vi "XPS_LTA_HS_Jogger.vi"(4 "Axis 2":string="Group3", 5 "Axis 1":string="Group2", 7 "Controller Address":string="192.168.254.254") -> ()   [LabVIEW 2016]
panel:
  in  "stop 2":bool
  in  "Refresh Time\n(msec)":u32=100 min=50 max=10000 step=1
  out "Axis 2 position":dbl format="%.10f"
  out "Axis 1 position":dbl format="%.10f"
  out "Axis 2 Status":string
  out "Axis 1 Status":string
  in  "Velocity (slow)\nmm/s":dbl=1.0 min=0.0 max=5.0
  in  "Velocity (fast)\nmm/s":dbl=5.0 min=0.0 max=5.0
  in  "Fast motion parameter":T1={"Velocity (units/s)"=5.0, "Acceleration (units/s²)"=20.0} {"Acceleration (units/s²)" format="%.6f"; "Velocity (units/s)" format="%.6f"}
  in  "Axis 2 Positive fast":bool
  in  "Axis 2 Positive":bool
  in  "Axis 2 negative fast":bool
  in  "Axis 2 negative":bool
  in  "Axis 1 Positive fast":bool
  in  "Axis 1 Positive":bool
  in  "Axis 1 negative fast":bool
  in  "Axis 1 negative":bool
  in  "Slow motion parameter":T1={"Velocity (units/s)"=1.0, "Acceleration (units/s²)"=20.0} {"Acceleration (units/s²)" format="%.6f"; "Velocity (units/s)" format="%.6f"}
  in  "stop":bool
  # "1"
  # "2"
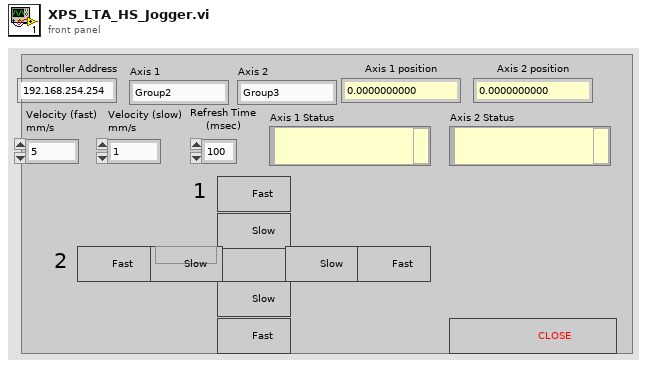
[diagram p1: front panel]
types:
  T1 = cluster{"Velocity (units/s)":dbl, "Acceleration (units/s²)":dbl}
  T2 = cluster{"connection TCP":refnum<k5>, "LogTo File":bool, "Log File refnum":refnum<file>, "no error if error log":bool}
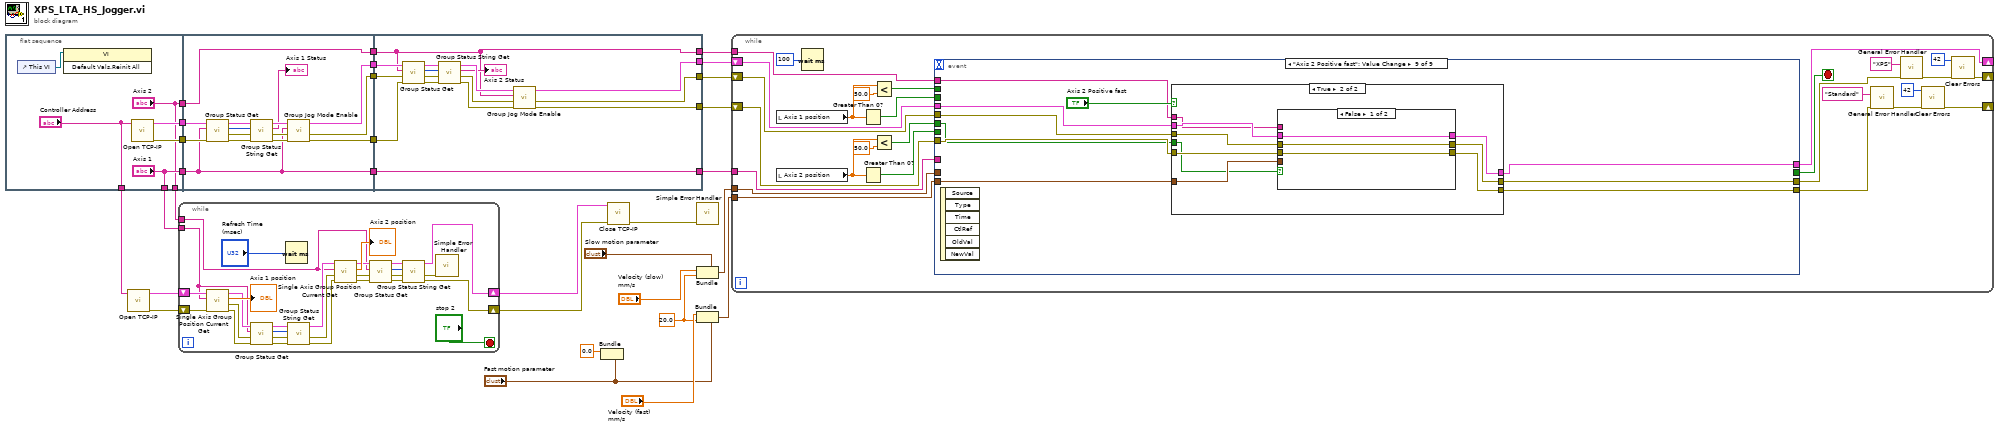
[diagram p0: block diagram]
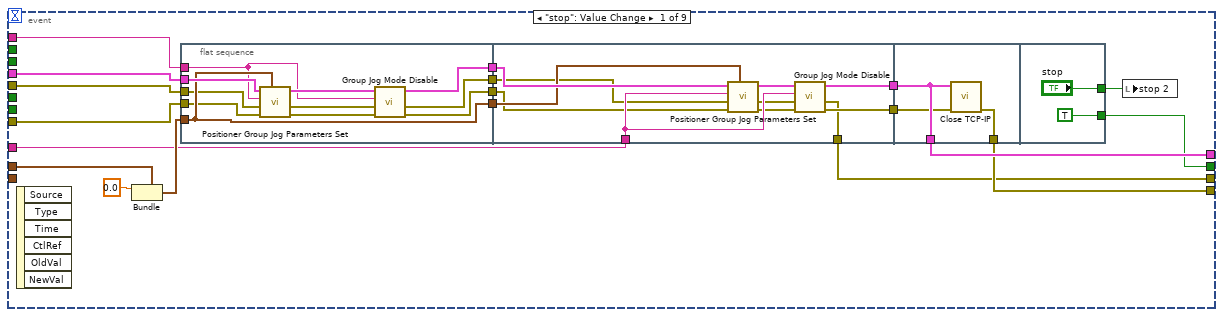
[diagram p2: hidden frame]
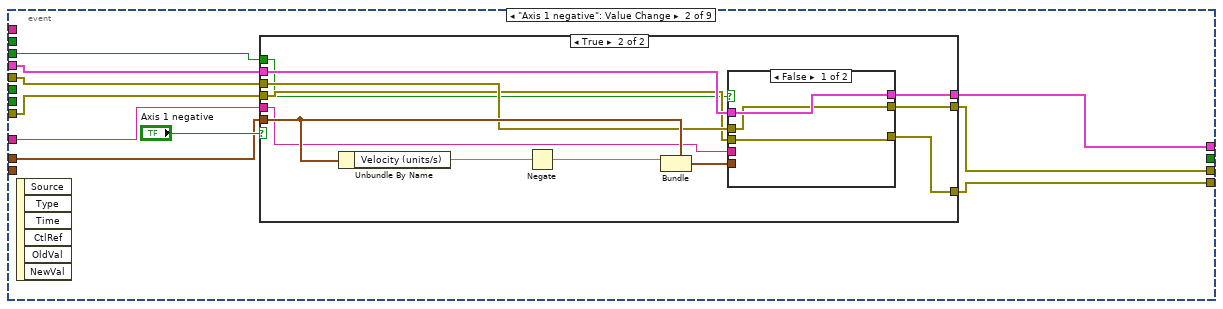
[diagram p3: hidden frame]
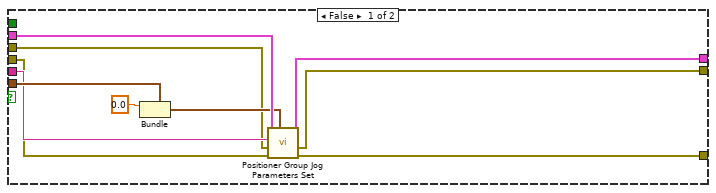
[diagram p4: hidden frame]
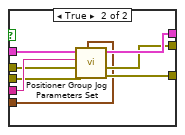
[diagram p5: hidden frame]
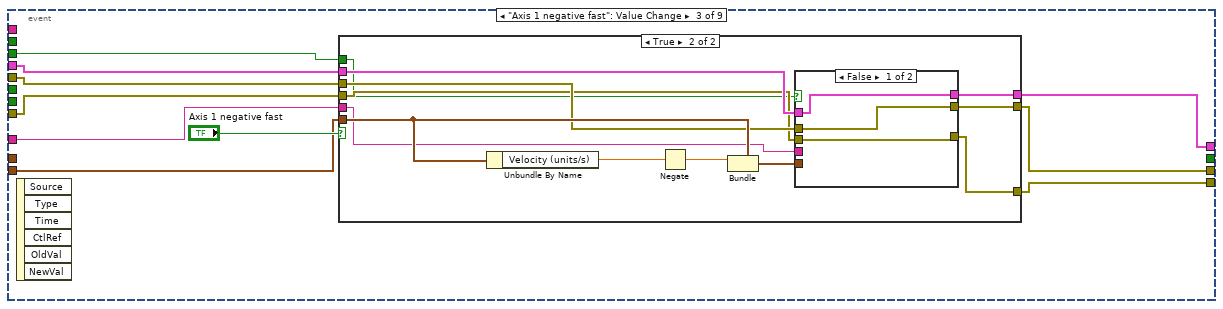
[diagram p6: hidden frame]
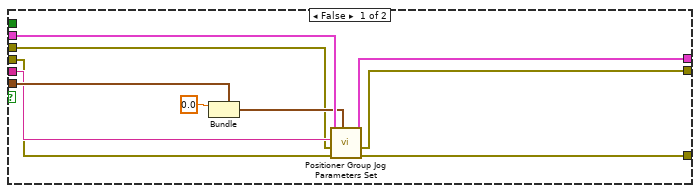
[diagram p7: hidden frame]
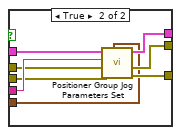
[diagram p8: hidden frame]
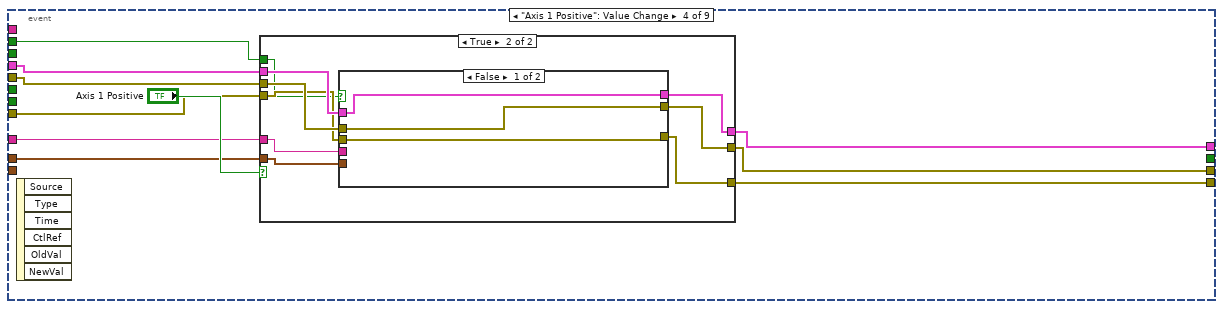
[diagram p9: hidden frame]
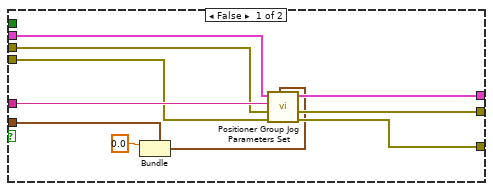
[diagram p10: hidden frame]
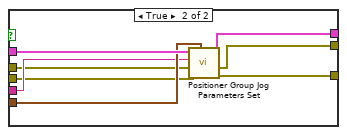
[diagram p11: hidden frame]
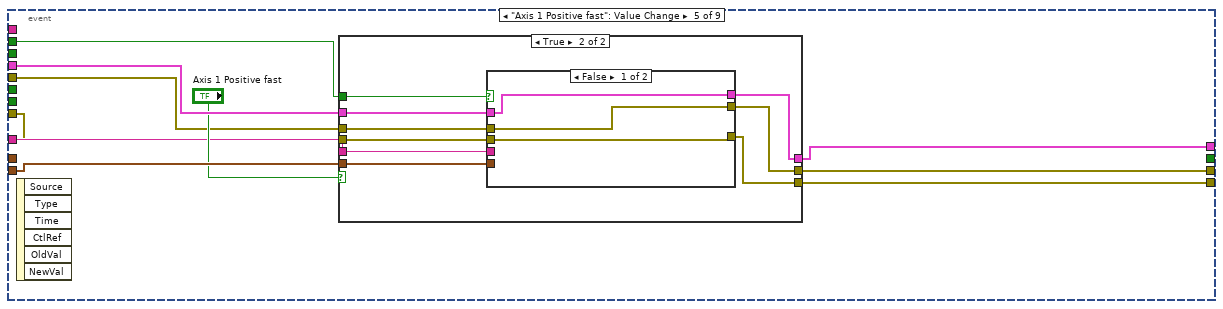
[diagram p12: hidden frame]
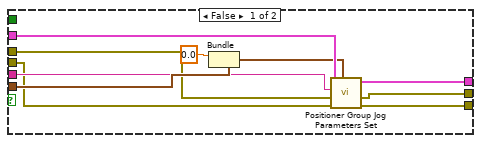
[diagram p13: hidden frame]
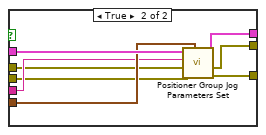
[diagram p14: hidden frame]
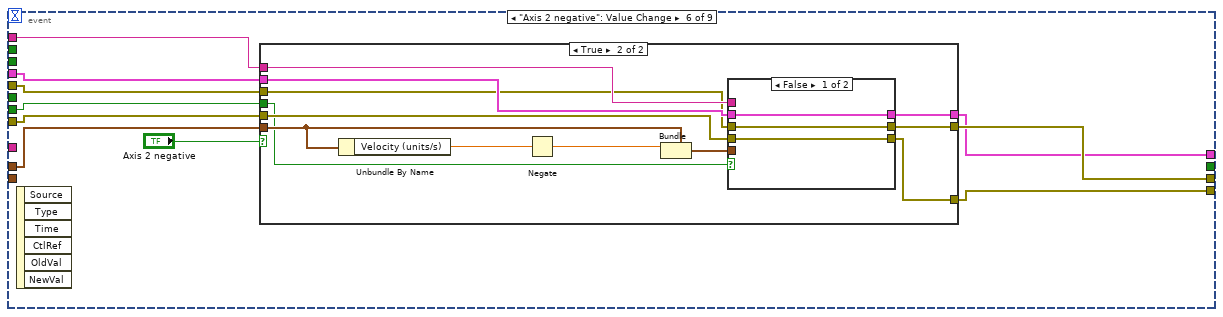
[diagram p15: hidden frame]
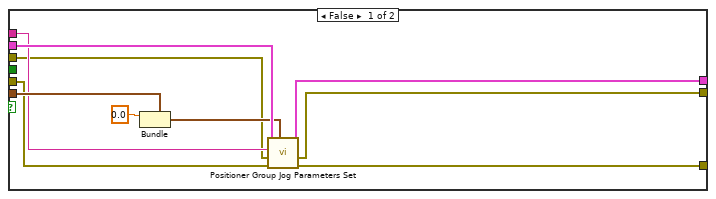
[diagram p16: hidden frame]
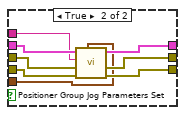
[diagram p17: hidden frame]
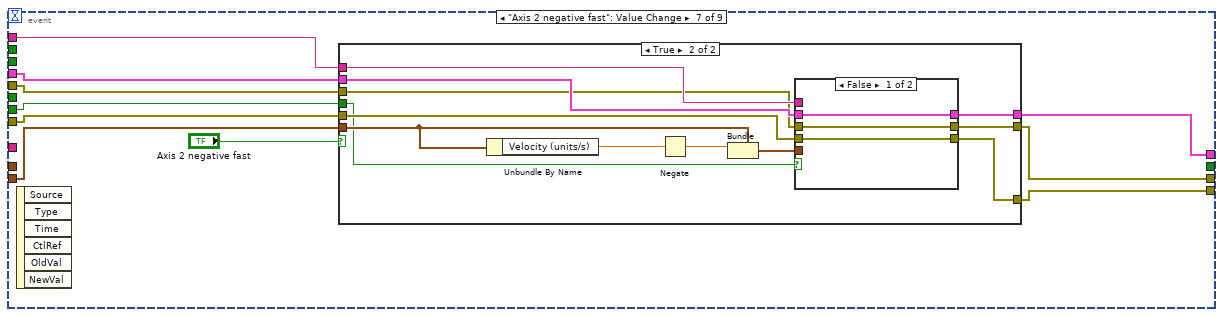
[diagram p18: hidden frame]
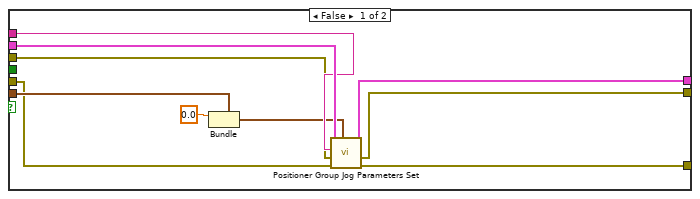
[diagram p19: hidden frame]
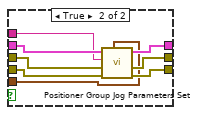
[diagram p20: hidden frame]
diagram:
  w22 = 20.0 ("Acceleration (units/s²)")
  n1 = flat-sequence {
    tunnel: ["Axis 1"] -> w19
    tunnel: [w35] -> w18
    tunnel: [w34] -> w17
    tunnel: ["Axis 2"] -> w16
    tunnel: ["Controller Address"] -> w10
    tunnel: ["Axis 1"] -> w5
    tunnel: ["Axis 2"] -> w4
    tunnel: [w51] -> w30
    tunnel: [w50] -> w29
    tunnel: [w49] -> w28
    tunnel: w19 -> [w37]
    tunnel: w18 -> [w44]
    tunnel: w17 -> [w43]
    tunnel: w16 -> [w38]
    tunnel: [w38] -> w15
    tunnel: [w37] -> w13
    tunnel: w30 -> [w64]
    tunnel: w29 -> [w58]
    tunnel: w28 -> [w59]
    tunnel: w15 -> [w53]
    tunnel: w13 -> [w54]
    tunnel: [w57] -> w2
    tunnel: [w56] -> w14
    tunnel: [w54] -> w11
    tunnel: [w53] -> w12
    tunnel: [w52] -> w1
    frame #0 {
      n2 = control-ref of="This VI"() -> (w36:refnum<vi>)
      n3 = invoke class="VI" method="Default Vals.Reinit All"(reference=w36) -> ()  [unwired: 2 in, 3 out]
      n4 = call <userlib>:"Open TCP-IP.vi"("IP address"="Controller Address") -> ("error out"=w35:errorcluster, "Connection ID"=w34:T2)  [unwired: 5 in, 4 out]
    }
    frame #1 {
      n5 = call <userlib>:"Group Status Get.vi"("error in (no error)"=w44, "Group Name (250 c max)"=w37, "connection ID in"=w43) -> ("error out"=w47:errorcluster, "XPS error out"=w48:errorcluster, "Status"=w46:i32, "connection ID out"=w42:T2)  [unwired: 5 in]
      n6 = call <userlib>:"Group Status String Get.vi"("error in (no error)"=w47, "XPS error in (no error)"=w48, "Status #"=w46, "connection ID in"=w42) -> ("error out"=w41:errorcluster, "XPS error out"=w40:errorcluster, "Group Status String"=→"Axis 1 Status":string, "connection ID out"=w45:T2)  [unwired: 4 in]
      n7 = call <userlib>:"Group Jog Mode Enable.vi"("error in (no error)"=w41, "XPS error in (no error)"=w40, "Group Name (250 c max)"=w37, "connection ID in"=w45) -> ("error out"=w49:errorcluster, "XPS error out"=w50:errorcluster, "connection ID out"=w51:T2)  [unwired: 5 in]
    }
    frame #2 {
      n8 = call <userlib>:"Group Status Get.vi"("error in (no error)"=w59, "XPS error in (no error)"=w58, "Group Name (250 c max)"=w53, "connection ID in"=w64) -> ("error out"=w66:errorcluster, "XPS error out"=w67:errorcluster, "Status"=w65:i32, "connection ID out"=w63:T2)  [unwired: 4 in]
      n9 = call <userlib>:"Group Status String Get.vi"("error in (no error)"=w66, "XPS error in (no error)"=w67, "Status #"=w65, "connection ID in"=w63) -> ("error out"=w61:errorcluster, "XPS error out"=w60:errorcluster, "Group Status String"=→"Axis 2 Status":string, "connection ID out"=w62:T2)  [unwired: 4 in]
      n10 = call <userlib>:"Group Jog Mode Enable.vi"("error in (no error)"=w61, "XPS error in (no error)"=w60, "Group Name (250 c max)"=w53, "connection ID in"=w62) -> ("error out"=w52:errorcluster, "XPS error out"=w57:errorcluster, "connection ID out"=w56:T2)  [unwired: 5 in]
    }
  }
  n11 = call <userlib>:"Open TCP-IP.vi"("IP address"=w10) -> ("error out"=w8:errorcluster, "Connection ID"=w9:T2)  [unwired: 5 in, 4 out]
  n12 = while {
    shift-right: [w70] -> w7
    shift-left: w9 -> [w95]
    shift-right: [w69] -> w6
    shift-left: w8 -> [w94]
    tunnel: w5 -> [w86]
    tunnel: w4 -> [w73]
    stop <- "stop 2" stop-if-true
    n13 = call <userlib>:"Single Axis Group Position Current Get.vi"("error in (no error)"=w94, "SingleAxis Group  Name (250 c max)"=w86, "connection ID in"=w95) -> ("error out"=w85:errorcluster, "XPS error out"=w84:errorcluster, "Current Position (units)"=→"Axis 1 position":dbl, "connection ID out"=w89:T2)  [unwired: 5 in]
    n14 = call <userlib>:"Group Status Get.vi"("error in (no error)"=w85, "XPS error in (no error)"=w84, "Group Name (250 c max)"=w86, "connection ID in"=w89) -> ("error out"=w82:errorcluster, "XPS error out"=w83:errorcluster, "Status"=w87:i32, "connection ID out"=w88:T2)  [unwired: 4 in]
    n15 = Wait (ms)(milliseconds to wait="Refresh Time\n(msec)") -> ()  [unwired: 1 out]
    n16 = call <userlib>:"Group Status String Get.vi"("error in (no error)"=w82, "XPS error in (no error)"=w83, "Status #"=w87, "connection ID in"=w88) -> ("error out"=w79:errorcluster, "XPS error out"=w80:errorcluster, "connection ID out"=w81:T2)  [unwired: 4 in, 1 out]
    n17 = call <userlib>:"Single Axis Group Position Current Get.vi"("error in (no error)"=w79, "XPS error in (no error)"=w80, "SingleAxis Group  Name (250 c max)"=w73, "connection ID in"=w81) -> ("error out"=w76:errorcluster, "XPS error out"=w77:errorcluster, "Current Position (units)"=→"Axis 2 position":dbl, "connection ID out"=w78:T2)  [unwired: 4 in]
    n18 = call <userlib>:"Group Status Get.vi"("error in (no error)"=w76, "XPS error in (no error)"=w77, "Group Name (250 c max)"=w73, "connection ID in"=w78) -> ("error out"=w74:errorcluster, "XPS error out"=w75:errorcluster, "Status"=w71:i32, "connection ID out"=w72:T2)  [unwired: 4 in]
    n19 = call <userlib>:"Group Status String Get.vi"("error in (no error)"=w74, "XPS error in (no error)"=w75, "Status #"=w71, "connection ID in"=w72) -> ("error out"=w69:errorcluster, "XPS error out"=w68:errorcluster, "connection ID out"=w70:T2)  [unwired: 4 in, 1 out]
    n20 = call <vilib>:"Simple Error Handler.vi"("error in (no error)"=w68) -> ()  [unwired: 4 in, 5 out]
  }
  n21 = Bundle(cluster="Fast motion parameter", "Velocity (units/s)"=0.0) -> ()  [unwired: 1 in, 1 out]
  n22 = call <userlib>:"Close TCP-IP.vi"("error in (no error)"=w6, "connection ID in"=w7) -> ("Error out"=w3:errorcluster)  [unwired: 9 in]
  n23 = call <vilib>:"Simple Error Handler.vi"("error in (no error)"=w3) -> ()  [unwired: 4 in, 5 out]
  n24 = Bundle(cluster="Slow motion parameter", "Velocity (units/s)"="Velocity (slow)\nmm/s", "Acceleration (units/s²)"=w22) -> (w24:T1)
  n25 = Bundle(cluster="Fast motion parameter", "Velocity (units/s)"="Velocity (fast)\nmm/s", "Acceleration (units/s²)"=w22) -> (w27:T1)
  n26 = while {
    shift-right: [w122] -> _
    shift-left: w14 -> [w123]
    tunnel: w27 -> [w121]
    tunnel: w24 -> [w120]
    tunnel: w12 -> [w119]
    tunnel: w11 -> [w118]
    shift-right: [w96] -> _
    shift-left: w1 -> [w107]
    shift-right: [w99] -> _
    shift-left: w2 -> [w108]
    stop <- w114 stop-if-true
    n27 = local read "Axis 1 position"() -> (w110:dbl)
    n28 = local read "Axis 2 position"() -> (w109:dbl)
    n29 = Wait (ms)(milliseconds to wait=u32 100) -> ()  [unwired: 1 out]
    n30 = Greater Than 0?(x=w110) -> (x > 0?=w106:bool)
    n31 = Greater Than 0?(x=w109) -> (x > 0?=w104:bool)
    n32 = Less?(x=w110, y=50.0) -> (x < y?=w105:bool)
    n33 = Less?(x=w109, y=50.0) -> (x < y?=w103:bool)
    n34 = event shown="[8] \"Axis 2 Positive fast\": Value Change" {
      selector: _ -> [_ _ _ _ _ _ _ _ _]
      dyn-events: _ -> [_ _ _ _ _ _ _ _ _]
      timeout: _ -> [_ _ _ _ _ _ _ _ _]
      tunnel: [w125 w175 w218 w261 w304 w341 w383 w426 w466] -> w115
      tunnel: w123 -> [w142 w178 w221 w264 w305 w343 w386 w429 w470]
      tunnel: [w141 w177 w220 w263 w302 w340 w385 w428 w468] -> w122
      tunnel: [w124 w176 w219 w262 w303 w342 w384 w427 w467] -> w116
      tunnel: w121 -> [_ _ w217 _ w301 _ w387 _ w469]
      tunnel: w120 -> [w137 w174 _ w260 _ w344 _ w430 _]
      tunnel: w119 -> [w134 _ _ _ _ w339 w382 w425 w465]
      tunnel: w118 -> [w133 w173 w216 w259 w299 _ _ _ _]
      tunnel: [w132 _ _ _ _ _ _ _ _] -> w114
      tunnel: w108 -> [w130 w172 w215 w258 w298 w338 w381 w424 w464]
      tunnel: w107 -> [w126 w171 w214 w257 w297 w337 w380 w423 w463]
      tunnel: w106 -> [_ w170 w213 _ _ _ _ _ _]
      tunnel: w105 -> [_ _ _ w256 w296 _ _ _ _]
      tunnel: w104 -> [_ _ _ _ _ w336 w379 _ _]
      tunnel: w103 -> [_ _ _ _ _ _ _ w422 w462]
      event "stop": Value Change {
        n35 = event-data() -> ()  [unwired: 1 in, 6 out]
        n36 = Bundle(cluster=w137, "Velocity (units/s)"=0.0) -> (w136:T1)  [unwired: 1 in]
        n37 = flat-sequence {
          tunnel: w142 -> [w152]
          tunnel: [w151] -> w139
          tunnel: w136 -> [w150]
          tunnel: [w150] -> w135
          tunnel: w134 -> [w149]
          tunnel: w130 -> [w148]
          tunnel: [w146] -> w129
          tunnel: [w145] -> w127
          tunnel: w126 -> [w143]
          tunnel: [w162] -> w140
          tunnel: w139 -> [w164]
          tunnel: w135 -> [w161]
          tunnel: w133 -> [w160]
          tunnel: w129 -> [w159]
          tunnel: [w157] -> w128
          tunnel: w127 -> [w155]
          tunnel: [w154] -> w124
          tunnel: [w167] -> w141
          tunnel: w140 -> [w167]
          tunnel: w128 -> [w166]
          tunnel: [w165] -> w125
          tunnel: [TRUE] -> w132
          tunnel: ["stop"] -> w131
          frame #0 {
            n38 = call <userlib>:"Positioner Group Jog Parameters Set.vi"("Group Jog parameters"=w150, "error in (no error)"=w143, "XPS error in (no error)"=w148, "Positioner Name (250 c max)"=w149, "connection ID in"=w152) -> ("error out"=w144:errorcluster, "XPS error out"=w147:errorcluster, "connection ID out"=w153:T2)  [unwired: 4 in]
            n39 = call <userlib>:"Group Jog Mode Disable.vi"("error in (no error)"=w144, "XPS error in (no error)"=w147, "Group Name (250 c max)"=w149, "connection ID in"=w153) -> ("error out"=w145:errorcluster, "XPS error out"=w146:errorcluster, "connection ID out"=w151:T2)  [unwired: 5 in]
          }
          frame #1 {
            n40 = call <userlib>:"Positioner Group Jog Parameters Set.vi"("Group Jog parameters"=w161, "error in (no error)"=w155, "XPS error in (no error)"=w159, "Positioner Name (250 c max)"=w160, "connection ID in"=w164) -> ("error out"=w156:errorcluster, "XPS error out"=w158:errorcluster, "connection ID out"=w163:T2)  [unwired: 4 in]
            n41 = call <userlib>:"Group Jog Mode Disable.vi"("error in (no error)"=w156, "XPS error in (no error)"=w158, "Group Name (250 c max)"=w160, "connection ID in"=w163) -> ("error out"=w157:errorcluster, "XPS error out"=w154:errorcluster, "connection ID out"=w162:T2)  [unwired: 5 in]
          }
          frame #2 {
            n42 = call <userlib>:"Close TCP-IP.vi"("error in (no error)"=w166, "connection ID in"=w167) -> ("Error out"=w165:errorcluster)  [unwired: 9 in]
          }
          frame #3 {
          }
        }
        n43 = local write "stop 2"(w131) -> ()
      }
      event "Axis 1 negative": Value Change {
        n44 = event-data() -> ()  [unwired: 1 in, 6 out]
        n45 = case shown="True" "Axis 1 negative" {
          tunnel: w178 -> [w188 w201]
          tunnel: [w187 w199] -> w177
          tunnel: [w186 w198] -> w176
          tunnel: [w185 w197] -> w175
          tunnel: w174 -> [w189 w200]
          tunnel: w173 -> [w184 w196]
          tunnel: w172 -> [w181 w192]
          tunnel: w171 -> [w180 w191]
          tunnel: w170 -> [_ w190]
          frame False {
            n46 = Bundle(cluster=w189, "Velocity (units/s)"=0.0) -> (w182:T1)  [unwired: 1 in]
            n47 = call <userlib>:"Positioner Group Jog Parameters Set.vi"("Group Jog parameters"=w182, "error in (no error)"=w180, "XPS error in (no error)"=w181, "Positioner Name (250 c max)"=w184, "connection ID in"=w188) -> ("error out"=w185:errorcluster, "XPS error out"=w186:errorcluster, "connection ID out"=w187:T2)  [unwired: 4 in]
          }
          frame True {
            n48 = Unbundle By Name(w200) -> ("Velocity (units/s)"=w195:dbl)
            n49 = Negate(x=w195) -> (-x=w194:dbl)
            n50 = Bundle(cluster=w200, "Velocity (units/s)"=w194) -> (w193:T1)  [unwired: 1 in]
            n51 = case shown="False" w190 {
              tunnel: w201 -> [w204 w212]
              tunnel: [w204 w211] -> w199
              tunnel: [w203 w210] -> w198
              tunnel: [w202 w209] -> w197
              tunnel: w196 -> [_ w208]
              tunnel: w193 -> [_ w207]
              tunnel: w192 -> [w203 w206]
              tunnel: w191 -> [w202 w205]
              frame False {
              }
              frame True {
                n52 = call <userlib>:"Positioner Group Jog Parameters Set.vi"("Group Jog parameters"=w207, "error in (no error)"=w205, "XPS error in (no error)"=w206, "Positioner Name (250 c max)"=w208, "connection ID in"=w212) -> ("error out"=w209:errorcluster, "XPS error out"=w210:errorcluster, "connection ID out"=w211:T2)  [unwired: 4 in]
              }
            }
          }
        }
      }
      event "Axis 1 negative fast": Value Change {
        n53 = event-data() -> ()  [unwired: 1 in, 6 out]
        n54 = case shown="True" "Axis 1 negative fast" {
          tunnel: w221 -> [w231 w244]
          tunnel: [w230 w242] -> w220
          tunnel: [w229 w241] -> w219
          tunnel: [w228 w240] -> w218
          tunnel: w217 -> [w232 w243]
          tunnel: w216 -> [w227 w239]
          tunnel: w215 -> [w224 w235]
          tunnel: w214 -> [w223 w234]
          tunnel: w213 -> [_ w233]
          frame False {
            n55 = Bundle(cluster=w232, "Velocity (units/s)"=0.0) -> (w225:T1)  [unwired: 1 in]
            n56 = call <userlib>:"Positioner Group Jog Parameters Set.vi"("Group Jog parameters"=w225, "error in (no error)"=w223, "XPS error in (no error)"=w224, "Positioner Name (250 c max)"=w227, "connection ID in"=w231) -> ("error out"=w228:errorcluster, "XPS error out"=w229:errorcluster, "connection ID out"=w230:T2)  [unwired: 4 in]
          }
          frame True {
            n57 = Unbundle By Name(w243) -> ("Velocity (units/s)"=w238:dbl)
            n58 = Negate(x=w238) -> (-x=w237:dbl)
            n59 = Bundle(cluster=w243, "Velocity (units/s)"=w237) -> (w236:T1)  [unwired: 1 in]
            n60 = case shown="False" w233 {
              tunnel: w244 -> [w245 w255]
              tunnel: [w245 w254] -> w242
              tunnel: [w246 w253] -> w241
              tunnel: [w247 w252] -> w240
              tunnel: w239 -> [_ w251]
              tunnel: w236 -> [_ w250]
              tunnel: w235 -> [w246 w249]
              tunnel: w234 -> [w247 w248]
              frame False {
              }
              frame True {
                n61 = call <userlib>:"Positioner Group Jog Parameters Set.vi"("Group Jog parameters"=w250, "error in (no error)"=w248, "XPS error in (no error)"=w249, "Positioner Name (250 c max)"=w251, "connection ID in"=w255) -> ("error out"=w252:errorcluster, "XPS error out"=w253:errorcluster, "connection ID out"=w254:T2)  [unwired: 4 in]
              }
            }
          }
        }
      }
      event "Axis 1 Positive": Value Change {
        n62 = event-data() -> ()  [unwired: 1 in, 6 out]
        n63 = case shown="True" "Axis 1 Positive" {
          tunnel: w264 -> [w275 w284]
          tunnel: [w273 w282] -> w263
          tunnel: [w272 w281] -> w262
          tunnel: [w271 w280] -> w261
          tunnel: w260 -> [w274 w283]
          tunnel: w259 -> [w270 w279]
          tunnel: w258 -> [w267 w278]
          tunnel: w257 -> [w266 w277]
          tunnel: w256 -> [_ w276]
          frame False {
            n64 = Bundle(cluster=w274, "Velocity (units/s)"=0.0) -> (w268:T1)  [unwired: 1 in]
            n65 = call <userlib>:"Positioner Group Jog Parameters Set.vi"("Group Jog parameters"=w268, "error in (no error)"=w266, "XPS error in (no error)"=w267, "Positioner Name (250 c max)"=w270, "connection ID in"=w275) -> ("error out"=w271:errorcluster, "XPS error out"=w272:errorcluster, "connection ID out"=w273:T2)  [unwired: 4 in]
          }
          frame True {
            n66 = case shown="False" w276 {
              tunnel: w284 -> [w285 w295]
              tunnel: w283 -> [_ w294]
              tunnel: [w285 w293] -> w282
              tunnel: [w287 w292] -> w281
              tunnel: [w286 w291] -> w280
              tunnel: w279 -> [_ w290]
              tunnel: w278 -> [w287 w289]
              tunnel: w277 -> [w286 w288]
              frame False {
              }
              frame True {
                n67 = call <userlib>:"Positioner Group Jog Parameters Set.vi"("Group Jog parameters"=w294, "error in (no error)"=w288, "XPS error in (no error)"=w289, "Positioner Name (250 c max)"=w290, "connection ID in"=w295) -> ("error out"=w291:errorcluster, "XPS error out"=w292:errorcluster, "connection ID out"=w293:T2)  [unwired: 4 in]
              }
            }
          }
        }
      }
      event "Axis 1 Positive fast": Value Change {
        n68 = event-data() -> ()  [unwired: 1 in, 6 out]
        n69 = case shown="True" "Axis 1 Positive fast" {
          tunnel: w305 -> [w315 w324]
          tunnel: [w311 w320] -> w304
          tunnel: [w312 w321] -> w303
          tunnel: [w313 w322] -> w302
          tunnel: w301 -> [w314 w323]
          tunnel: w299 -> [w310 w319]
          tunnel: w298 -> [w307 w317]
          tunnel: w297 -> [w306 w318]
          tunnel: w296 -> [_ w316]
          frame False {
            n70 = Bundle(cluster=w314, "Velocity (units/s)"=0.0) -> (w308:T1)  [unwired: 1 in]
            n71 = call <userlib>:"Positioner Group Jog Parameters Set.vi"("Group Jog parameters"=w308, "error in (no error)"=w306, "XPS error in (no error)"=w307, "Positioner Name (250 c max)"=w310, "connection ID in"=w315) -> ("error out"=w311:errorcluster, "XPS error out"=w312:errorcluster, "connection ID out"=w313:T2)  [unwired: 4 in]
          }
          frame True {
            n72 = case shown="False" w316 {
              tunnel: w324 -> [w325 w335]
              tunnel: w323 -> [_ w334]
              tunnel: [w325 w333] -> w322
              tunnel: [w327 w332] -> w321
              tunnel: [w326 w331] -> w320
              tunnel: w319 -> [_ w330]
              tunnel: w318 -> [w326 w329]
              tunnel: w317 -> [w327 w328]
              frame False {
              }
              frame True {
                n73 = call <userlib>:"Positioner Group Jog Parameters Set.vi"("Group Jog parameters"=w334, "error in (no error)"=w329, "XPS error in (no error)"=w328, "Positioner Name (250 c max)"=w330, "connection ID in"=w335) -> ("error out"=w331:errorcluster, "XPS error out"=w332:errorcluster, "connection ID out"=w333:T2)  [unwired: 4 in]
              }
            }
          }
        }
      }
      event "Axis 2 negative": Value Change {
        n74 = event-data() -> ()  [unwired: 1 in, 6 out]
        n75 = case shown="True" "Axis 2 negative" {
          tunnel: w344 -> [w354 w367]
          tunnel: w343 -> [w355 w366]
          tunnel: [w352 w364] -> w342
          tunnel: [w351 w363] -> w341
          tunnel: [w353 w365] -> w340
          tunnel: w339 -> [w350 w362]
          tunnel: w338 -> [w347 w358]
          tunnel: w337 -> [w346 w357]
          tunnel: w336 -> [_ w356]
          frame False {
            n76 = Bundle(cluster=w354, "Velocity (units/s)"=0.0) -> (w348:T1)  [unwired: 1 in]
            n77 = call <userlib>:"Positioner Group Jog Parameters Set.vi"("Group Jog parameters"=w348, "error in (no error)"=w346, "XPS error in (no error)"=w347, "Positioner Name (250 c max)"=w350, "connection ID in"=w355) -> ("error out"=w351:errorcluster, "XPS error out"=w352:errorcluster, "connection ID out"=w353:T2)  [unwired: 4 in]
          }
          frame True {
            n78 = Unbundle By Name(w367) -> ("Velocity (units/s)"=w361:dbl)
            n79 = Negate(x=w361) -> (-x=w360:dbl)
            n80 = Bundle(cluster=w367, "Velocity (units/s)"=w360) -> (w359:T1)  [unwired: 1 in]
            n81 = case shown="False" w356 {
              tunnel: w366 -> [w370 w378]
              tunnel: [w370 w377] -> w365
              tunnel: [w369 w376] -> w364
              tunnel: [w368 w375] -> w363
              tunnel: w362 -> [_ w374]
              tunnel: w359 -> [_ w373]
              tunnel: w358 -> [w369 w372]
              tunnel: w357 -> [w368 w371]
              frame False {
              }
              frame True {
                n82 = call <userlib>:"Positioner Group Jog Parameters Set.vi"("Group Jog parameters"=w373, "error in (no error)"=w371, "XPS error in (no error)"=w372, "Positioner Name (250 c max)"=w374, "connection ID in"=w378) -> ("error out"=w375:errorcluster, "XPS error out"=w376:errorcluster, "connection ID out"=w377:T2)  [unwired: 4 in]
              }
            }
          }
        }
      }
      event "Axis 2 negative fast": Value Change {
        n83 = event-data() -> ()  [unwired: 1 in, 6 out]
        n84 = case shown="True" "Axis 2 negative fast" {
          tunnel: w387 -> [w397 w410]
          tunnel: w386 -> [w398 w409]
          tunnel: [w396 w408] -> w385
          tunnel: [w395 w407] -> w384
          tunnel: [w394 w406] -> w383
          tunnel: w382 -> [w393 w405]
          tunnel: w381 -> [w390 w401]
          tunnel: w380 -> [w389 w400]
          tunnel: w379 -> [_ w399]
          frame False {
            n85 = Bundle(cluster=w397, "Velocity (units/s)"=0.0) -> (w391:T1)  [unwired: 1 in]
            n86 = call <userlib>:"Positioner Group Jog Parameters Set.vi"("Group Jog parameters"=w391, "error in (no error)"=w389, "XPS error in (no error)"=w390, "Positioner Name (250 c max)"=w393, "connection ID in"=w398) -> ("error out"=w394:errorcluster, "XPS error out"=w395:errorcluster, "connection ID out"=w396:T2)  [unwired: 4 in]
          }
          frame True {
            n87 = Unbundle By Name(w410) -> ("Velocity (units/s)"=w404:dbl)
            n88 = Negate(x=w404) -> (-x=w403:dbl)
            n89 = Bundle(cluster=w410, "Velocity (units/s)"=w403) -> (w402:T1)  [unwired: 1 in]
            n90 = case shown="False" w399 {
              tunnel: w409 -> [w413 w421]
              tunnel: [w413 w420] -> w408
              tunnel: [w412 w419] -> w407
              tunnel: [w411 w418] -> w406
              tunnel: w405 -> [_ w417]
              tunnel: w402 -> [_ w416]
              tunnel: w401 -> [w412 w415]
              tunnel: w400 -> [w411 w414]
              frame False {
              }
              frame True {
                n91 = call <userlib>:"Positioner Group Jog Parameters Set.vi"("Group Jog parameters"=w416, "error in (no error)"=w414, "XPS error in (no error)"=w415, "Positioner Name (250 c max)"=w417, "connection ID in"=w421) -> ("error out"=w418:errorcluster, "XPS error out"=w419:errorcluster, "connection ID out"=w420:T2)  [unwired: 4 in]
              }
            }
          }
        }
      }
      event "Axis 2 Positive": Value Change {
        n92 = event-data() -> ()  [unwired: 1 in, 6 out]
        n93 = case shown="True" "Axis 2 Positive" {
          tunnel: w430 -> [w440 w449]
          tunnel: w429 -> [w441 w450]
          tunnel: [w439 w448] -> w428
          tunnel: [w438 w447] -> w427
          tunnel: [w437 w446] -> w426
          tunnel: w425 -> [w436 w445]
          tunnel: w424 -> [w432 w444]
          tunnel: w423 -> [w433 w443]
          tunnel: w422 -> [_ w442]
          frame False {
            n94 = Bundle(cluster=w440, "Velocity (units/s)"=0.0) -> (w434:T1)  [unwired: 1 in]
            n95 = call <userlib>:"Positioner Group Jog Parameters Set.vi"("Group Jog parameters"=w434, "error in (no error)"=w433, "XPS error in (no error)"=w432, "Positioner Name (250 c max)"=w436, "connection ID in"=w441) -> ("error out"=w437:errorcluster, "XPS error out"=w438:errorcluster, "connection ID out"=w439:T2)  [unwired: 4 in]
          }
          frame True {
            n96 = case shown="False" w442 {
              tunnel: w450 -> [w453 w461]
              tunnel: w449 -> [_ w460]
              tunnel: [w453 w459] -> w448
              tunnel: [w452 w458] -> w447
              tunnel: [w451 w457] -> w446
              tunnel: w445 -> [_ w456]
              tunnel: w444 -> [w452 w455]
              tunnel: w443 -> [w451 w454]
              frame False {
              }
              frame True {
                n97 = call <userlib>:"Positioner Group Jog Parameters Set.vi"("Group Jog parameters"=w460, "error in (no error)"=w454, "XPS error in (no error)"=w455, "Positioner Name (250 c max)"=w456, "connection ID in"=w461) -> ("error out"=w457:errorcluster, "XPS error out"=w458:errorcluster, "connection ID out"=w459:T2)  [unwired: 4 in]
              }
            }
          }
        }
      }
      event "Axis 2 Positive fast": Value Change {
        n98 = event-data() -> ()  [unwired: 1 in, 6 out]
        n99 = case shown="True" "Axis 2 Positive fast" {
          tunnel: w470 -> [w481 w490]
          tunnel: w469 -> [w480 w489]
          tunnel: [w479 w486] -> w468
          tunnel: [w478 w487] -> w467
          tunnel: [w477 w488] -> w466
          tunnel: w465 -> [w476 w485]
          tunnel: w464 -> [w472 w484]
          tunnel: w463 -> [w473 w483]
          tunnel: w462 -> [_ w482]
          frame False {
            n100 = Bundle(cluster=w480, "Velocity (units/s)"=0.0) -> (w474:T1)  [unwired: 1 in]
            n101 = call <userlib>:"Positioner Group Jog Parameters Set.vi"("Group Jog parameters"=w474, "error in (no error)"=w473, "XPS error in (no error)"=w472, "Positioner Name (250 c max)"=w476, "connection ID in"=w481) -> ("error out"=w477:errorcluster, "XPS error out"=w478:errorcluster, "connection ID out"=w479:T2)  [unwired: 4 in]
          }
          frame True {
            n102 = case shown="False" w482 {
              tunnel: w490 -> [w493 w501]
              tunnel: w489 -> [_ w500]
              tunnel: [w491 w499] -> w488
              tunnel: [w492 w498] -> w487
              tunnel: [w493 w497] -> w486
              tunnel: w485 -> [_ w496]
              tunnel: w484 -> [w492 w495]
              tunnel: w483 -> [w491 w494]
              frame False {
              }
              frame True {
                n103 = call <userlib>:"Positioner Group Jog Parameters Set.vi"("Group Jog parameters"=w500, "error in (no error)"=w494, "XPS error in (no error)"=w495, "Positioner Name (250 c max)"=w496, "connection ID in"=w501) -> ("error out"=w499:errorcluster, "XPS error out"=w498:errorcluster, "connection ID out"=w497:T2)  [unwired: 4 in]
              }
            }
          }
        }
      }
    }
    n104 = call <vilib>:"General Error Handler.vi"("[error source] (\" \")"="Standard" ("[error source] (\" \")"), "error in (no error)"=w115) -> ("error out"=w97:errorcluster)  [unwired: 9 in, 4 out]
    n105 = call <vilib>:"General Error Handler.vi"("[error source] (\" \")"="XPS" ("[error source] (\" \")"), "error in (no error)"=w116) -> ("error out"=w113:errorcluster)  [unwired: 9 in, 4 out]
    n106 = call <vilib>:"Clear Errors.vi"("error in (no error)"=w97, "specific error code to clear (0: all)"=42 ("y")) -> ("error out"=w96:errorcluster)  [unwired: 4 in, 1 out]
    n107 = call <vilib>:"Clear Errors.vi"("error in (no error)"=w113, "specific error code to clear (0: all)"=42 ("y")) -> ("error out"=w99:errorcluster)  [unwired: 4 in, 1 out]
  }
